vi "CRYRub & Buzz Loudness.vi"(8 "Version":i32, 9 "s[k]":dbl[](array[numeric]), 10 "E2[k]":dbl[](array[numeric]), 11 "Ethres[k]":dbl[](array[numeric])) -> (1 "Ntotal":dbl, 3 "N[k]":dbl[](array[numeric]))   [LabVIEW 2013]
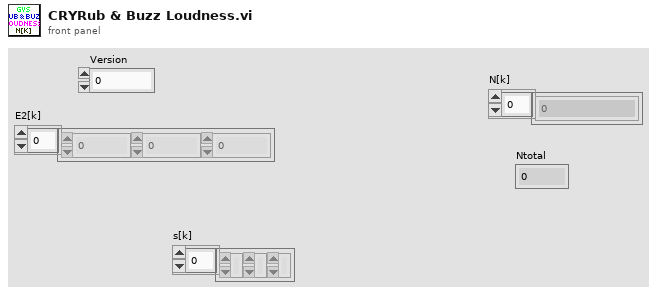
[diagram p1: front panel]
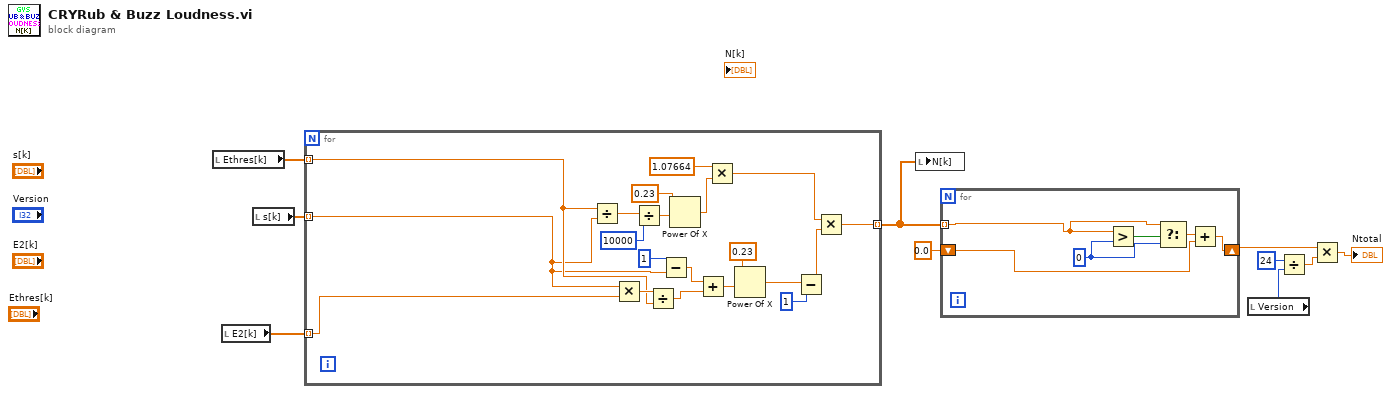
[diagram p0: block diagram]
diagram:
  n1 = local read "Ethres[k]"() -> (w3:dbl[])
  n2 = local read "E2[k]"() -> (w2:dbl[])
  n3 = local read "s[k]"() -> (w4:dbl[])
  n4 = for {
    tunnel: [w21] -> w1 mode=indexing
    tunnel: w3 -> [w15] mode=indexing
    tunnel: w4 -> [w14] mode=indexing
    tunnel: w2 -> [w11] mode=indexing
    n5 = Divide(x=w15, y=w14) -> (x/y=w24:dbl)
    n6 = Multiply ("Multiply.vi")(x=w14, y=w11) -> (x*y=w27:dbl)
    n7 = Divide(x=w24, y=10000) -> (x/y=w16:dbl)
    n8 = Divide(x=w27, y=w15) -> (x/y=w19:dbl)
    n9 = Subtract ("Subtract.vi")(x=1, y=w14) -> (x-y=w18:dbl)
    n10 = Power Of X ("Power Of X.vi")(1:w16, 2:0.23) -> (0:w13:dbl)
    n11 = Add ("Add.vi")(x=w18, y=w19) -> (x+y=w12:dbl)
    n12 = Multiply ("Multiply.vi")(x=1.07664, y=w13) -> (x*y=w22:dbl)
    n13 = Power Of X ("Power Of X.vi")(1:w12, 2:0.23) -> (0:w17:dbl)
    n14 = Subtract ("Subtract.vi")(x=w17, y=1) -> (x-y=w20:dbl)
    n15 = Multiply ("Multiply.vi")(x=w22, y=w20) -> (x*y=w21:dbl)
  }
  n16 = local write "N[k]"(w1) -> ()
  n17 = for {
    shift-right: [w33] -> w10
    shift-left: 0.0 -> [w32]
    tunnel: w1 -> [w31] mode=indexing
    w35 = 0
    n18 = Greater?(x=w31, y=w35) -> (0:w36:bool)
    n19 = Select(t=w31, s=w36, f=w35) -> (s? t:f=w34:dbl)
    n20 = Add(x=w34, y=w32) -> (x+y=w33:dbl)
  }
  n21 = local read "Version"() -> (w6:i32)
  n22 = Divide(x=24, y=w6) -> (x/y=w8:dbl)
  n23 = Multiply(x=w10, y=w8) -> (x*y=→"Ntotal":dbl)
